vi "Test2.vi"() -> ()   [LabVIEW 2020]
uses:
  Classes/KD Tree Double/KD Tree Double.lvclass
  E:/Labview/LV 2020/Libs/flann/Classes/KD Tree/KD Tree.lvclass
  Classes/KD Tree Double/Create KD Tree Double.vi
  Classes/KD Tree Double/Find Nearest Neighbors Index Double.vi
  Classes/KD Tree/KD Tree.lvclass
  E:/Labview/LV 2020/Libs/flann/Classes/KD Tree Double/KD Tree Double.lvclass
panel:
  out "Ref 2":u64
  out "Ref":u64
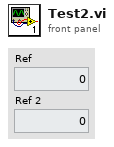
[diagram p1: front panel]
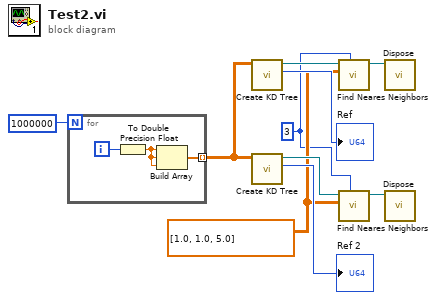
[diagram p0: block diagram]
diagram:
  w1 = 3 ("Max Neighbors")
  w2 = dbl[][] [[1.0, 1.0, 5.0]] ("Points")
  n1 = for {
    N: 1000000 -> [_]
    tunnel: [w11] -> w9 mode=indexing
    i -> [w13]
    n2 = To Double Precision Float(number=w13) -> (double precision float=w12:dbl)
    n3 = Build Array(w12, w12, w12) -> (w11:dbl[])
  }
  n4 = call-poly "Create KD Tree.vi"("Points (Row-Vectors)"=w9) -> ("Ref"=→"Ref":u64, "KD Tree Double out"=w8:refnum<class "KD Tree Double.lvclass">)  [unwired: 8 in, 1 out]
  n5 = call-poly "Create KD Tree.vi"("Points (Row-Vectors)"=w9) -> ("Ref"=→"Ref 2":u64, "KD Tree Double out"=w4:refnum<class "KD Tree Double.lvclass">)  [unwired: 8 in, 1 out]
  n6 = call-poly "Find Neares Neighbors.vi"("#Neighbors"=w1, "Points"=w2, "KD Tree Double in"=w8) -> ("KD Tree Double out"=w5:refnum<class "KD Tree Double.lvclass">)  [unwired: 5 in, 3 out]
  n7 = call-poly "Find Neares Neighbors.vi"("#Neighbors"=w1, "Points"=w2, "KD Tree Double in"=w4) -> ("KD Tree Double out"=w3:refnum<class "KD Tree Double.lvclass">)  [unwired: 5 in, 3 out]
  n8 = call "Dispose.vi"("KD Tree in"=w5) -> ()  [unwired: 10 in, 1 out]
  n9 = call "Dispose.vi"("KD Tree in"=w3) -> ()  [unwired: 10 in, 1 out]
